vi "Example Tag Read.vi"() -> ()   [LabVIEW 2017]
uses:
  <vilib>/NI/Current Value Table/DataTypes/Array of Double_Read.vi
  <vilib>/NI/Current Value Table/Type to Enum.vi
  <vilib>/NI/Current Value Table/DataTypes/Array of Double_Type To Enum.vi
  <vilib>/NI/Current Value Table/FGVs/CVT Globals.vi
  <vilib>/NI/Current Value Table/FGVs/Tag Memory.vi
  <vilib>/NI/Current Value Table/Memory Block.vi
  <vilib>/NI/Current Value Table/DataTypes/Array of Double_Memory Block.vi
  <vilib>/NI/Current Value Table/Current Value Table.lvlib
panel:
  in  "stop":bool
  out "error out":errorcluster
  out "Value":dbl[](array[numeric])
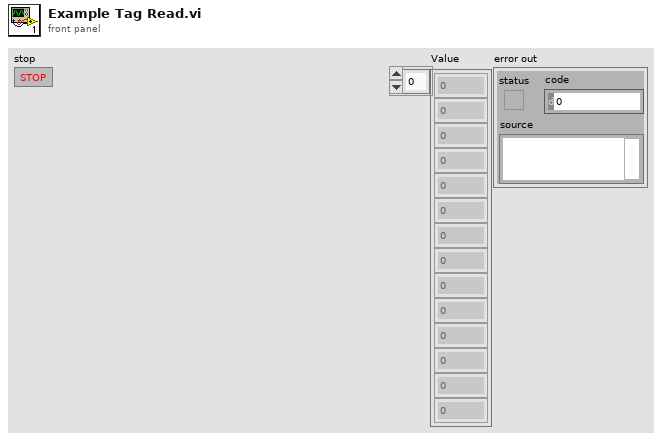
[diagram p1: front panel]
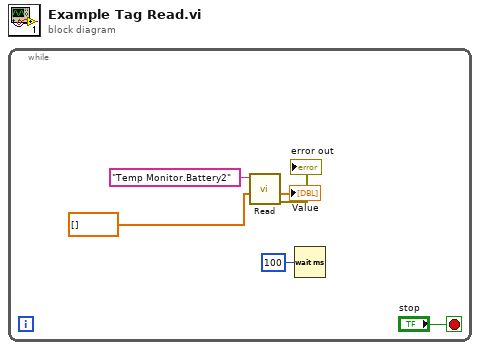
[diagram p0: block diagram]
diagram:
  n1 = while {
    stop <- "stop" stop-if-true
    n2 = call-poly <vilib>:"Read.vi"("Default"=dbl[] [], "Tag Name"="Temp Monitor.Battery2") -> ("error out"=→"error out":errorcluster, "Value"=→"Value":dbl[])  [unwired: 8 in]
    n3 = Wait (ms)(milliseconds to wait=u32 100) -> ()  [unwired: 1 out]
  }
